vi "niRFUtil MEAS Mean (complex array).vi"(7 "Complex Array":T1 format="%.2f") -> (8 "Mean":csg format="%.2f")   [LabVIEW 2015, in "niRFUtil.lvlib"]
doc: "(c) Copyright 2006, National Instruments, Inc. This VI may not be duplicated, sold, or distributed without written consent from National Instruments."
uses:
  niRFUtil.lvlib
  Includes/niRFUtil INC Complex Array.ctl
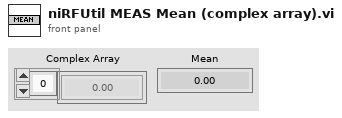
[diagram p1: front panel]
types:
  T1 = typedef "niRFUtil.lvlib/niRFUtil INC Complex Array.ctl" = csg[]
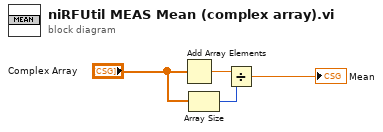
[diagram p0: block diagram]
diagram:
  n1 = Add Array Elements(numeric array="Complex Array") -> (sum=w1:csg)
  n2 = Array Size(array="Complex Array") -> (size(s)=w2:i32)
  n3 = Divide(x=w1, y=w2) -> (x/y=→"Mean":csg)
